vi "monochromatorCommandSetFactor.vi"(8 "error in":errorcluster, 9 "factor":dbl, 10 "grating":i32, 11 "monochromator":refnum<k24>) -> (0 "error out":errorcluster, 3 "monochromator":refnum<k24>)   [LabVIEW 2009]
doc: "Set Factor"
uses:
  C:/Users/anderson.chen/Desktop/Software Development/Cornerstone Series API (LV9)/Cornerstone DLL/Cornerstone.dll
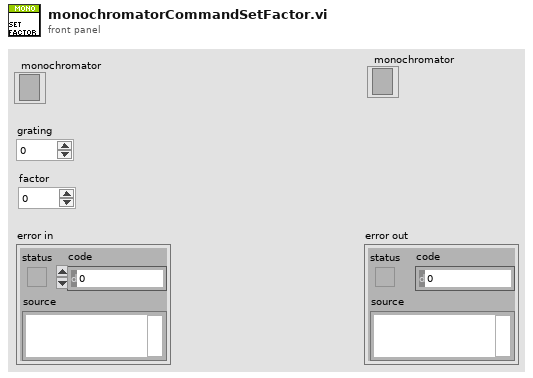
[diagram p1: front panel]
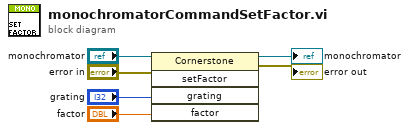
[diagram p0: block diagram]
diagram:
  n1 = invoke class="Cornerstone" method="setFactor"(reference="monochromator", error in="error in", "grating"="grating", "factor"="factor") -> (reference out=→"monochromator":refnum<k24>, error out=→"error out":errorcluster)  [unwired: 1 in, 3 out]
